vi "Select dll Path (SubVI).vi"(0 "Select dll Path":T1(ring)) -> (1 "dll Path out":path, 2 "error out":errorcluster)   [LabVIEW 2012]
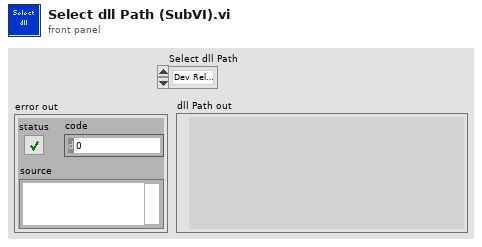
[diagram p1: front panel]
types:
  T1 = enum16{"Dev Release", "System", "Specify", "Empty"}
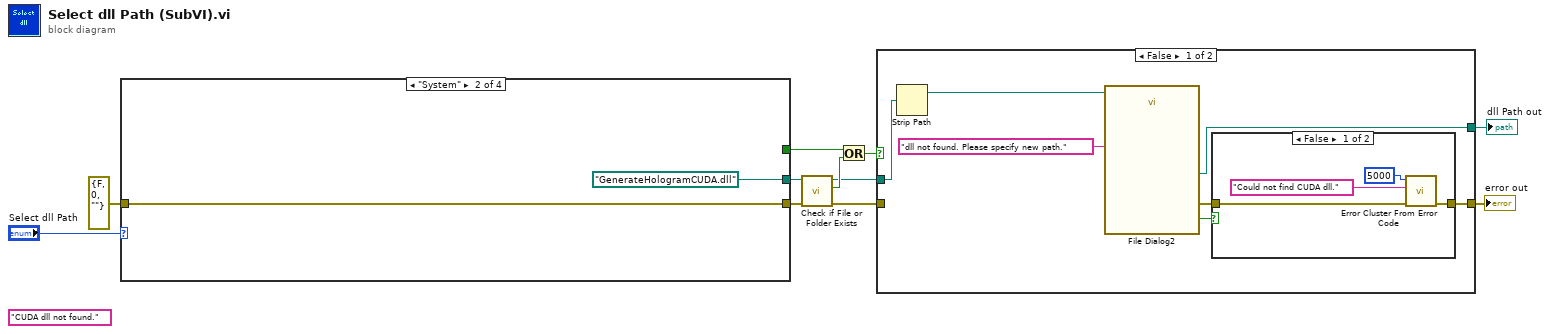
[diagram p0: block diagram]
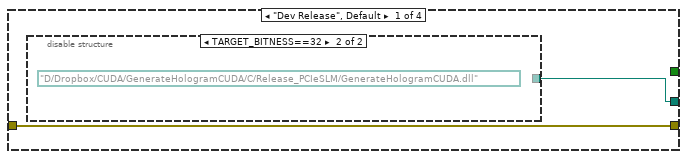
[diagram p4: hidden frame]
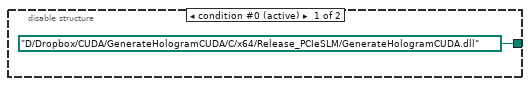
[diagram p5: hidden frame]
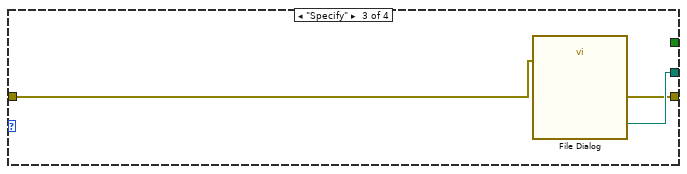
[diagram p6: hidden frame]
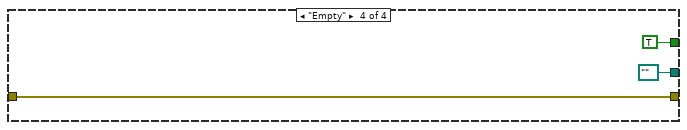
[diagram p7: hidden frame]
diagram:
  (unwired) "CUDA dll not found." ("error message (\"\")")
  n1 = case shown="\"System\"" "Select dll Path" {
    tunnel: [w13 path "GenerateHologramCUDA.dll" ("dll Path 2") w19 path "" ("dll Path 2")] -> w10
    tunnel: errorcluster {"status"=FALSE, "code"=0, "source"=""} ("error in (no error)") -> [w12 w15 w18 w21]
    tunnel: [w12 w15 w17 w21] -> w4
    tunnel: [_ _ _ TRUE ("x")] -> w2
    frame "Dev Release", Default {
      n2 = disable-structure shown="TARGET_BITNESS==32" {
        disable-tunnel: [path "D:/Dropbox/CUDA/GenerateHologramCUDA/C/x64/Release_PCIeSLM/GenerateHologramCUDA.dll" ("path in") _] -> w13
        frame condition #0 (active) {
        }
        frame condition #1 {
          (unwired) path "D:/Dropbox/CUDA/GenerateHologramCUDA/C/Release_PCIeSLM/GenerateHologramCUDA.dll" ("path in")
        }
      }
    }
    frame "System" {
    }
    frame "Specify" {
      n3 = call "File Dialog"("error in"=w18) -> ("selected path"=w19:path, "error out"=w17:errorcluster)  [unwired: 11 in, 2 out]
    }
    frame "Empty" {
    }
  }
  n4 = call <vilib>:"Check if File or Folder Exists.vi"("error in (no error)"=w4, "path"=w10) -> ("error out"=w6:errorcluster, "file or folder exists?"=w9:bool, "dup path"=w7:path)  [unwired: 7 in]
  n5 = Or(x=w2, y=w9) -> (x .or. y?=w3:bool)
  n6 = case shown="False" w3 {
    tunnel: [w28 w36] -> w8
    tunnel: w7 -> [w27 w36]
    tunnel: w6 -> [_ w35]
    tunnel: [w23 w35] -> w1
    frame False {
      n7 = Strip Path(path=w27) -> (stripped path=w26:path)  [unwired: 1 out]
      n8 = call "File Dialog2"("start path"=w26, "prompt"="dll not found. Please specify new path.") -> ("selected path"=w28:path, "exists"=w24:bool, "error out"=w25:errorcluster)  [unwired: 10 in, 1 out]
      n9 = case shown="False" w24 {
        tunnel: w25 -> [w33 w34]
        tunnel: [w32 w34] -> w23
        frame False {
          n10 = call <vilib>:"Error Cluster From Error Code.vi"("error in (no error)"=w33, "error message (\"\")"="Could not find CUDA dll." ("error message (\"\")"), "error code (0)"=5000) -> ("error out"=w32:errorcluster)  [unwired: 6 in]
        }
        frame True {
        }
      }
    }
    frame True {
    }
  }
  "dll Path out" <- w8
  "error out" <- w1
